vi "Actor Core.vi"(8 "error in":errorcluster, 11 "Particle Counter in":refnum<class "Particle Counter.lvclass">) -> (0 "error out":errorcluster, 3 "Actor out":refnum<class "Actor.lvclass">)   [LabVIEW 2023, in "Particle Counter.lvlib" / "Particle Counter.lvclass"]
doc: "(<B>Filename</B>: Actor Framework.lvlib:Actor.lvclass:Actor Core.vi)\n\nReceives messages to the actor, reacts to them, and initiates any error handling that may shut the actor down.\n\nDescendant classes may override this VI to append parallel tasks for the actor to complete while it handles messages. Overrides use the Call Parent Class Method node."
uses:
  Particle Counter.lvclass
  C:/Program Files/National Instruments/LabVIEW 2023/vi.lib/ActorFramework/Actor/Actor.lvclass
  <vilib>/ActorFramework/Actor/Actor.lvclass
  <vilib>/ActorFramework/Actor/Actor.lvclass/Actor.ctl
  <vilib>/ActorFramework/Message Enqueuer/Message Enqueuer.lvclass/Message Enqueuer.ctl
  Particle Counter.lvclass/Particle Counter.ctl
  Particle Counter Messages/Log Counts Msg/Log Counts Msg.lvclass/Log Counts Msg.ctl
  <vilib>/ActorFramework/Message Enqueuer/Init from Existing Queue.vi
  <vilib>/ActorFramework/Message Enqueuer/Enqueue.vi
  Particle Counter Messages/Log Counts Msg/Log Counts Msg.lvclass
  C:/Program Files/National Instruments/LabVIEW 2023/vi.lib/ActorFramework/Message/Message.lvclass
  Resources/GLOBAL/GLOBAL Time-critical.vi
  <vilib>/ActorFramework/Message Priority Queue/Priority Enqueue.vi
  <vilib>/ActorFramework/Message Enqueuer/Message Enqueuer.lvclass
  User Interface/Viewer/Viewer.lvlib
panel:
  in  "STOP":bool
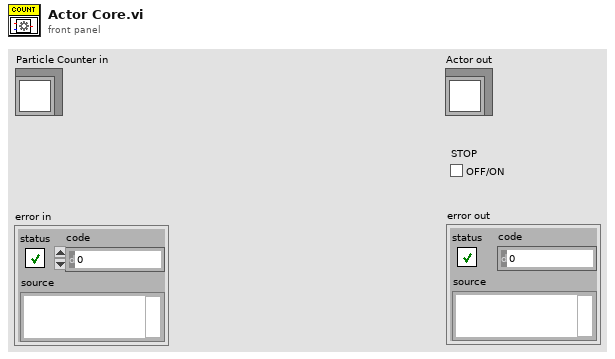
[diagram p1: front panel]
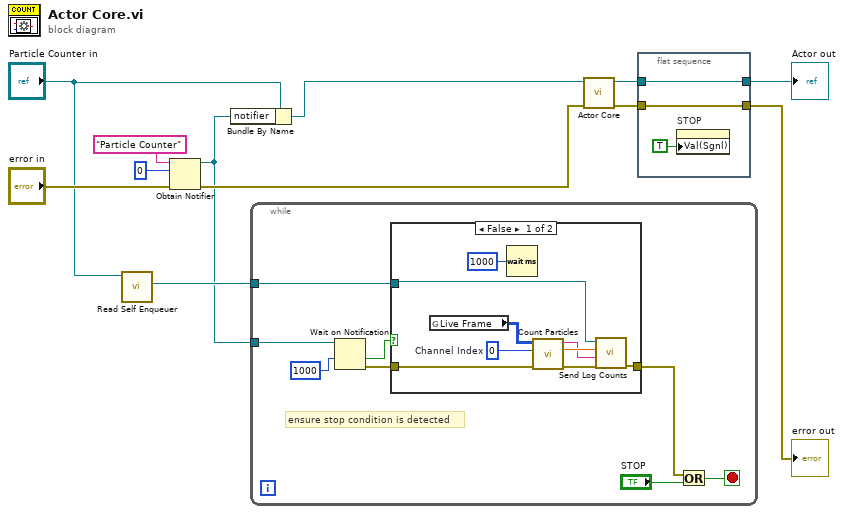
[diagram p0: block diagram]
diagram:
  n1 = call <vilib>:"Read Self Enqueuer.vi"("Actor"="Particle Counter in") -> ("Self Enqueuer"=w8:refnum<class "Message Enqueuer.lvclass">)  [unwired: 10 in]
  n2 = Obtain Notifier(name (unnamed)="Particle Counter", notification data type=0 ("Frame Number\n(starts with 1)"), error in (no error)="error in") -> (notifier out=w1:refnum<notifier>, error out=w4:errorcluster)  [unwired: 1 in, 1 out]
  n3 = Bundle By Name(cluster="Particle Counter in", "notifier"=w1) -> (w2:refnum<class "Particle Counter.lvclass">)
  n4 = while {
    tunnel: w8 -> [w13]
    tunnel: w1 -> [w17]
    stop <- w20 stop-if-true
    # "ensure stop condition is detected"
    n5 = Wait on Notification(notifier=w17, timeout in ms (-1)=1000) -> (timed out?=w15:bool, error out=w16:errorcluster)  [unwired: 2 in, 2 out]
    n6 = case shown="False" w15 {
      tunnel: [w24 w30] -> w18
      tunnel: w16 -> [w27 w30]
      tunnel: w13 -> [w26 _]
      frame False {
        w28 = u16 0  # Channel Index
        n7 = global read "GLOBAL Time-critical.vi" "Live Frame"() -> (w29:u16[][][])
        n8 = Wait (ms)(milliseconds to wait=u32 1000) -> ()  [unwired: 1 out]
        n9 = call "Count Particles.vi"("error in"=w27, "Channel Index"=w28, "Live Frame"=w29) -> ("error out"=w25:errorcluster, "Numeric"=w23:dbl, "String"=w22:string)  [unwired: 6 in]
        n10 = call "Send Log Counts.vi"("error in (no error)"=w25, "Message"=w22, "Counts"=w23, "Message Enqueuer"=w26) -> ("error out"=w24:errorcluster)  [unwired: 6 in, 1 out]
      }
      frame True {
      }
    }
    n11 = Or(x=w18, y="STOP") -> (x .or. y?=w20:bool)
  }
  n12 = call-parent "Actor Core.vi"("error in"=w4, "Actor in"=w2) -> ("error out"=w10:errorcluster, "Actor out"=w12:refnum<class "Actor.lvclass">)  [unwired: 8 in]
  n13 = flat-sequence {
    tunnel: w12 -> [w33]
    tunnel: [w33] -> w11
    tunnel: w10 -> [w32]
    tunnel: [w32] -> w9
    frame #0 {
      n14 = property on="STOP" class="Bool (strict)"("Val(Sgnl)"=TRUE ("Value (Signaling)")) -> ()  [unwired: 2 in, 2 out]
    }
  }
  "error out" <- w9
  "Actor out" <- w11
